vi "Launcher.vi"   [LabVIEW 2020]
uses:
  actor/GUI/VG-VNA_GUI/VG-VNA_GUI/VG-VNA_GUI.lvclass
  C:/Program Files (x86)/National Instruments/LabVIEW 2020/vi.lib/ActorFramework/Actor/Actor.lvclass
  <vilib>/ActorFramework/Actor/Actor.lvclass
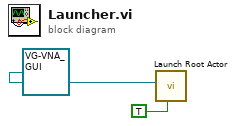
[diagram p0: block diagram]
diagram:
  n1 = call <vilib>:"Launch Root Actor.vi"("Open Actor Core front panel? (F)"=TRUE, "Actor"=refnum<class "VG-VNA_GUI.lvclass"> refnum ("VG-VNA_GUI.lvlib:VG-VNA_GUI.lvclass")) -> ()  [unwired: 8 in, 2 out]
